vi "2dynamic.vi"() -> ()   [LabVIEW 2026]
panel:
  in  "stop":bool
  in  "OK Button 3":bool
  in  "OK Button 2":bool
  in  "OK Button":bool
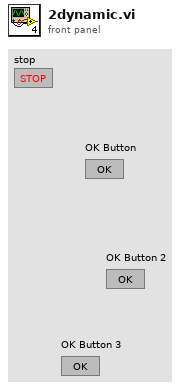
[diagram p1: front panel]
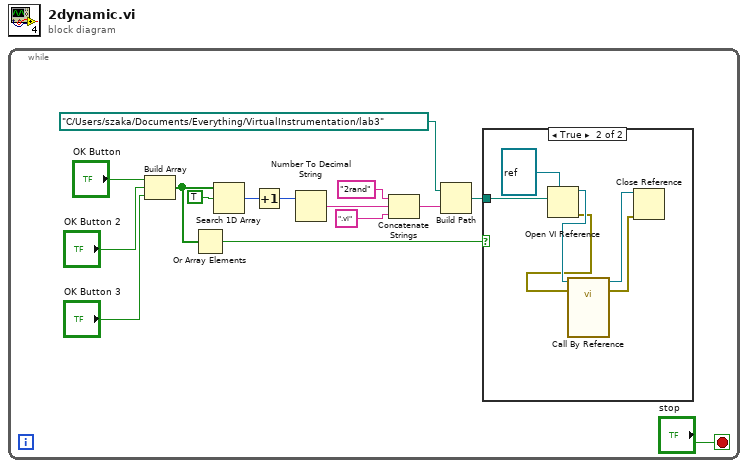
[diagram p0: block diagram]
diagram:
  n1 = while {
    stop <- "stop" stop-if-true
    n2 = Build Array("OK Button", "OK Button 2", "OK Button 3") -> (w4:bool[])
    n3 = Or Array Elements(Boolean array=w4) -> (logical OR=w3:bool)
    n4 = Search 1D Array(1D array=w4, element=TRUE) -> (index of element=w11:i32)  [unwired: 1 in]
    n5 = Increment(x=w11) -> (x+1=w10:i32)
    n6 = Number To Decimal String(number=w10) -> (decimal integer string=w9:string)  [unwired: 1 in]
    n7 = Concatenate Strings("2rand" ("string"), w9, ".vi" ("string")) -> (w6:string)
    n8 = Build Path(base path=path "C:/Users/szaka/Documents/Everything/VirtualInstrumentation/lab3", name or relative path=w6) -> (appended path=w2:path)
    n9 = case shown="True" w3 {
      tunnel: w2 -> [_ w20]
      frame False {
      }
      frame True {
        n10 = Open VI Reference(type specifier VI Refnum (for type only)=refnum<vi> refnum, vi path=w20) -> (vi reference=w19:refnum<vi>, error out=w17:errorcluster)  [unwired: 4 in]
        n11 = call-by-ref "?"(reference=w19, error in=w17) -> (reference out=w18:refnum<vi>, error out=w16:errorcluster)  [unwired: 12 in]
        n12 = Close Reference(reference=w18, error in (no error)=w16) -> ()  [unwired: 1 out]
      }
    }
  }
